vi "WritingFirstLabViewProgram.vi"() -> ()   [LabVIEW 2018]
panel:
  out "String":string
  in  "OK Button":bool
  out "Waveform Chart":dbl(graph)
  out "Gauge":dbl(knob) scale=0.0..10.0
  in  "Knob":dbl(knob) scale=0.0..10.0
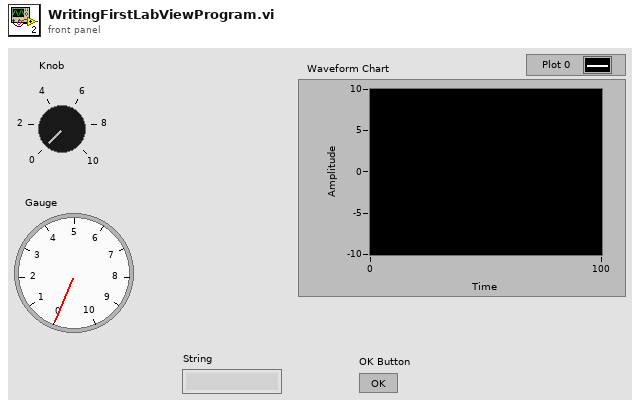
[diagram p1: front panel]
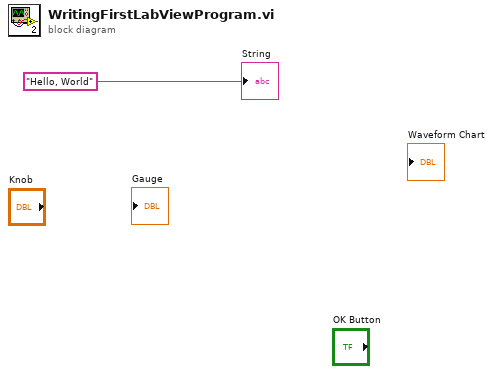
[diagram p0: block diagram]
diagram:
  "String" <- "Hello, World"
